vi "XNET.vi"(9 "Frame":T1 {"payload" format="%x"; "timestamp" format="%<%.7X\n%x>T"; "type" items=["CAN Data"=0, "CAN Remote"=1, "CAN Bus Error"=2, "CAN 2.0 Data"=8, "CAN FD Data"=16, "CAN FD+BRS Data"=24, "J1939 Data"=192, "Delay"=224, "Log Trigger"=225, "Start Trigger"=226]; "identifier" format="%x"}, 10 "ID":u32, 11 "DBC File":path) -> (2 "Human Readable DATA":string[][](array[string]), 3 "signal data":dbl[](array[numeric]) format="%.2f")   [LabVIEW 2025, in "CAN-LIN Raw Bus Capture UI.lvlib"]
uses:
  CAN-LIN Raw Bus Capture UI.lvlib
  <vilib>/xnet/xnet.llb/XNET Frame CAN.ctl
  <vilib>/xnet/xnet.llb/XNET Frame Type CAN.ctl
  <vilib>/xnet/xnet.llb/XNET Create Session (Conversion).vi
  <vilib>/xnet/xnet.llb/XNET Convert (Frame CAN to Signal).vi
  <resource>/objmgr/xnet.rc
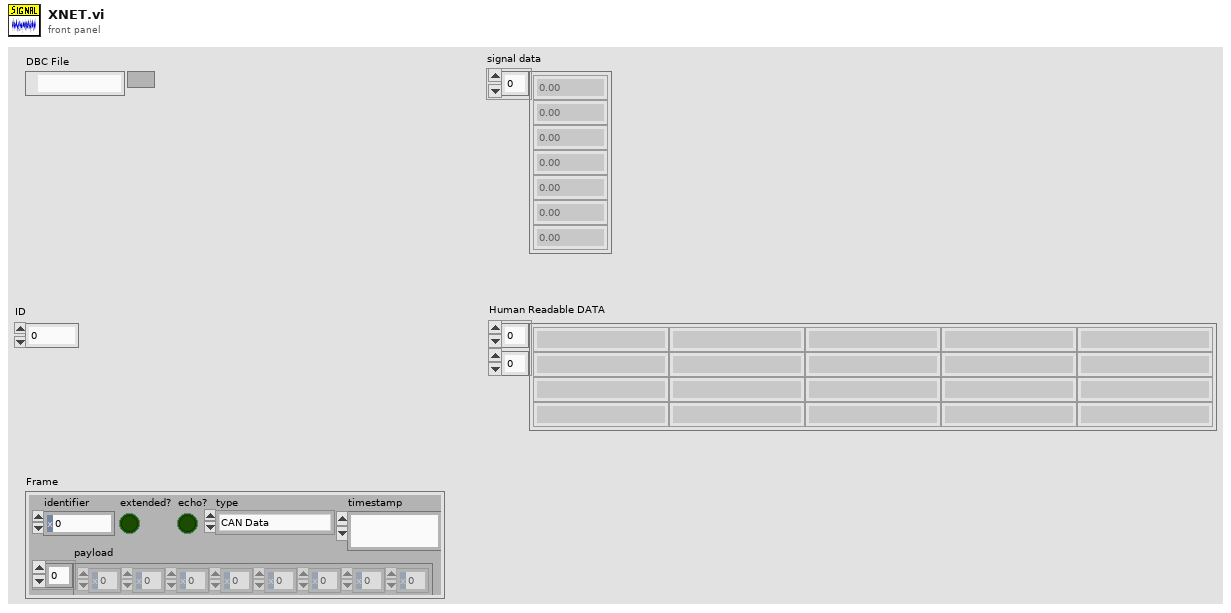
[diagram p1: front panel]
types:
  T1 = typedef "XNET Frame CAN.ctl" = cluster{"timestamp":timestamp, "payload":u8[], "identifier":u32, "type":T2, "extended?":bool, "echo?":bool}
  T2 = typedef "XNET Frame Type CAN.ctl" = u8
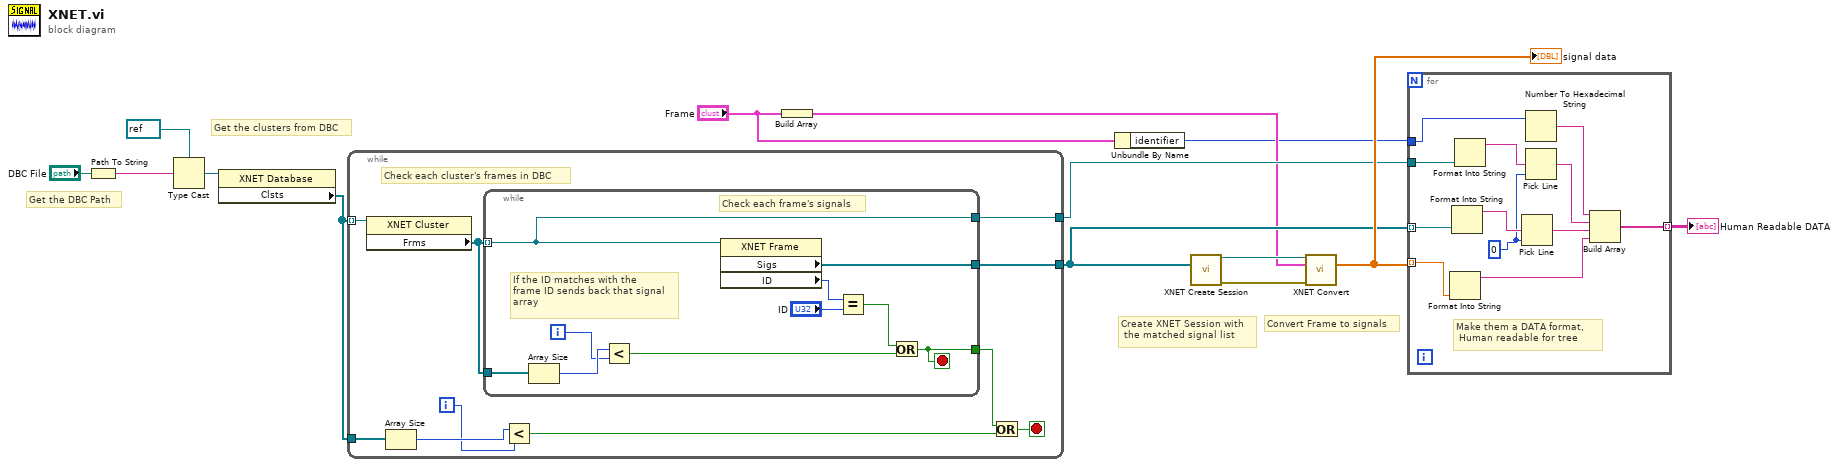
[diagram p0: block diagram]
diagram:
  # "Get the DBC Path"
  # "Convert Frame to signals"
  # "Create XNET Session with\n the matched signal list"
  # "Get the clusters from DBC"
  n1 = Path To String(path="DBC File") -> (string=w14:string)
  n2 = Type Cast(type=refnum<k21> refnum ("XNET Database"), x=w14) -> (*(type *) &x=w1:refnum<k21>)
  n3 = property class="XNET Database"(reference=w1) -> ("Clsts"=w2:refnum<k21>[])  [unwired: 1 in, 2 out]
  n4 = while {
    tunnel: w2 -> [w24] mode=indexing
    tunnel: [w23] -> w8
    tunnel: [w22] -> w6
    tunnel: w2 -> [w20]
    i -> [w15]
    stop <- w17 stop-if-true
    # "Check each cluster's frames in DBC"
    n5 = property class="XNET Cluster"(reference=w24) -> ("Frms"=w21:refnum<k21>[])  [unwired: 1 in, 2 out]
    n6 = Array Size(array=w20) -> (size(s)=w16:i32)
    n7 = while {
      tunnel: w21 -> [w31] mode=indexing
      tunnel: [w34] -> w23
      tunnel: [w31] -> w22
      tunnel: [w27] -> w19
      tunnel: w21 -> [w30]
      i -> [w25]
      stop <- w27 stop-if-true
      # "If the ID matches with the \nframe ID sends back that signal\narray"
      # "Check each frame's signals"
      n8 = Array Size(array=w30) -> (size(s)=w26:i32)
      n9 = Less?(x=w26, y=w25) -> (x < y?=w28:bool)
      n10 = property class="XNET Frame"(reference=w31) -> ("Sigs"=w34:refnum<k21>[], "ID"=w33:u32)  [unwired: 1 in, 2 out]
      n11 = Equal?(x=w33, y="ID") -> (x = y?=w29:bool)
      n12 = Or(x=w29, y=w28) -> (x .or. y?=w27:bool)
    }
    n13 = Less?(x=w16, y=w15) -> (x < y?=w18:bool)
    n14 = Or(x=w19, y=w18) -> (x .or. y?=w17:bool)
  }
  n15 = Build Array("Frame") -> (w5:T1[])
  n16 = Unbundle By Name("Frame") -> ("identifier"=w3:u32)
  n17 = call-poly <vilib>:"XNET Create Session.vi"("signal list"=w8) -> ("session out"=w10:refnum<k21>, "error out"=w11:errorcluster)  [unwired: 1 in, 12 out]
  n18 = call-poly <vilib>:"XNET Convert.vi"("session in"=w10, "frame data"=w5, "error in (no error)"=w11) -> ("signal data"=w9:dbl[])  [unwired: 12 out]
  "signal data" <- w9
  n19 = for {
    tunnel: w9 -> [w46] mode=indexing
    tunnel: w8 -> [w44] mode=indexing
    tunnel: [w43] -> w7 mode=indexing
    tunnel: w6 -> [w40]
    tunnel: w3 -> [w36]
    w38 = 0 ("line index")
    # "Make them a DATA format,\n Human readable for tree"
    n20 = Format Into String(w46) -> (resulting string=w45:string)  [unwired: 3 in, 1 out]
    n21 = Format Into String(w44) -> (resulting string=w42:string)  [unwired: 3 in, 1 out]
    n22 = Format Into String(w40) -> (resulting string=w39:string)  [unwired: 3 in, 1 out]
    n23 = Pick Line(multi-line string=w42, line index=w38) -> (output string=w41:string)  [unwired: 1 in]
    n24 = Number To Hexadecimal String(2:w36) -> (0:w35:string)  [unwired: 1 in]
    n25 = Pick Line(multi-line string=w39, line index=w38) -> (output string=w37:string)  [unwired: 1 in]
    n26 = Build Array(w35, w37, w41, w45) -> (w43:string[])
  }
  "Human Readable DATA" <- w7
